vi "UI--Update.vi"(8 "error in":errorcluster, 11 "Selector in":refnum<class "Selector.lvclass">) -> (0 "error out":errorcluster, 3 "Selector out":refnum<class "Selector.lvclass">)   [LabVIEW 2019, in "Selector.lvclass"]
uses:
  Selector.lvclass
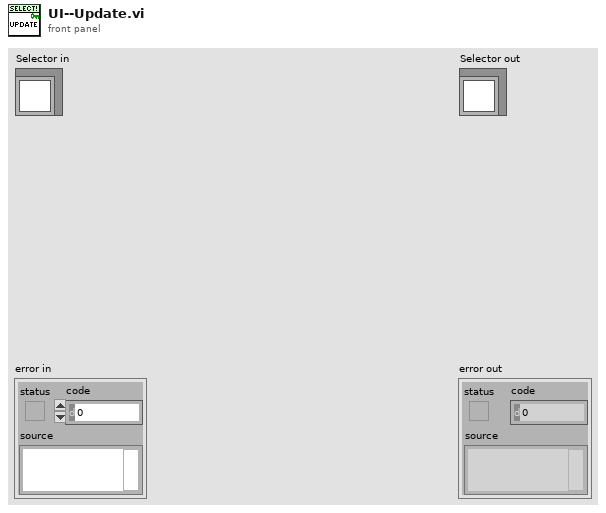
[diagram p1: front panel]
types:
  T1 = typedef "Selector.lvclass/Item.ctl" = cluster{"Name":string, "Group":string, "Enabled":bool}
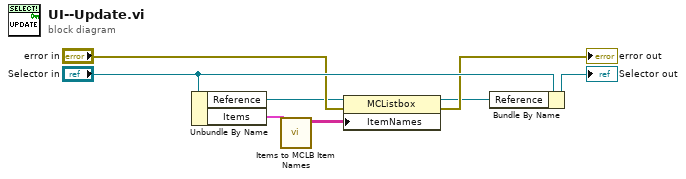
[diagram p0: block diagram]
diagram:
  n1 = Unbundle By Name("Selector in") -> ("Reference"=w2:refnum<vi>, "Items"=w7:T1[])
  n2 = call "Items to MCLB Item Names.vi"("Items"=w7) -> ("Item Names"=w8:string[][])  [unwired: 6 in]
  n3 = property class="MCListbox"(reference=w2, error in="error in", "ItemNames"=w8) -> (reference out=w1:refnum<vi>, error out=→"error out":errorcluster)
  n4 = Bundle By Name(cluster="Selector in", "Reference"=w1) -> (→"Selector out":refnum<class "Selector.lvclass">)
